vi "removeDuplicates.vi"(8 "error in (no error)":errorcluster, 10 "times":dbl[](array[numeric]) format="%#_18g", 11 "ScriptEventList in":refnum<class "ScriptEventList.lvclass">) -> (0 "error out":errorcluster, 2 "times out":dbl[](array[numeric]) format="%#_8g", 3 "ScriptEventList out":refnum<class "ScriptEventList.lvclass">)   [LabVIEW 2009, in "Tools.lvlib" / "Scripting.lvlib" / "ScriptEventList.lvclass"]
uses:
  ScriptEventList.lvclass
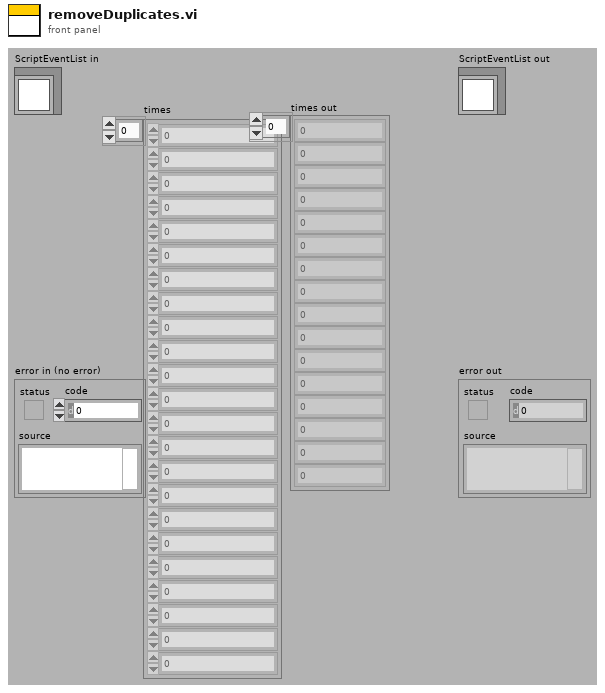
[diagram p1: front panel]
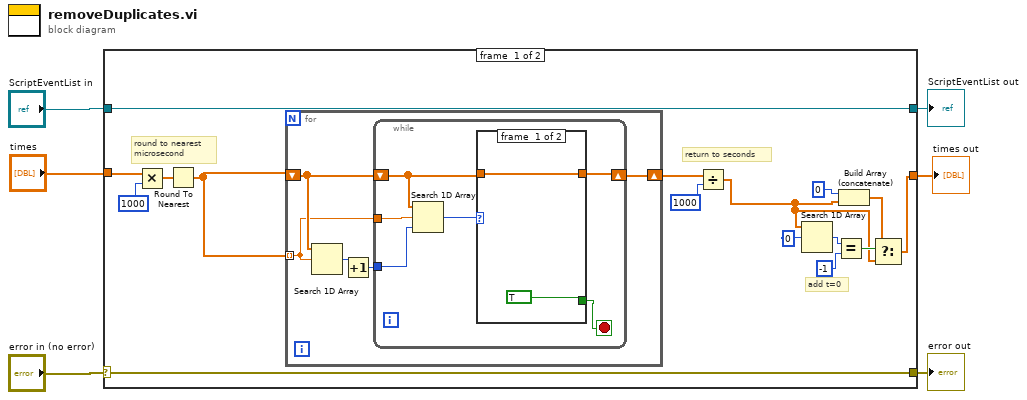
[diagram p0: block diagram]
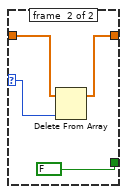
[diagram p2: hidden frame]
diagram:
  n1 = case shown="No Error" "error in (no error)" {
    selector: "error in (no error)" -> [w21 w41]
    tunnel: [w21 w41] -> w5
    tunnel: [w22 w40] -> w3
    tunnel: "ScriptEventList in" -> [w22 w40]
    tunnel: "times" -> [w20 _]
    tunnel: [w7 _] -> w1
    frame #0 {
      # "add t=0"
      # "return to seconds"
      # "round to nearest\nmicrosecond"
      n2 = Multiply(x=w20, y=1000) -> (x*y=w18:dbl[])
      n3 = Round To Nearest(number=w18) -> (nearest integer value=w17:dbl[])
      n4 = for {
        shift-right: [w27] -> w16
        shift-left: w17 -> [w24]
        tunnel: w17 -> [w23] mode=indexing
        n5 = Search 1D Array(1D array=w24, element=w23) -> (index of element=w26:i32)  [unwired: 1 in]
        n6 = Increment(x=w26) -> (x+1=w25:i32)
        n7 = while {
          shift-right: [w31] -> w27
          shift-left: w24 -> [w29]
          tunnel: w25 -> [w30]
          tunnel: w23 -> [w28]
          stop <- w32 stop-if-true
          n8 = Search 1D Array(1D array=w29, element=w28, start index (0)=w30) -> (index of element=w33:i32)
          n9 = case shown="-1" w33 {
            selector: w33 -> [_ w38]
            tunnel: [TRUE FALSE] -> w32
            tunnel: w29 -> [w34 w37]
            tunnel: [w34 w36] -> w31
            frame #0 {
            }
            frame #1 {
              n10 = Delete From Array(array=w37, index=w38) -> (array with subset deleted=w36:dbl[])  [unwired: 1 in, 1 out]
            }
          }
        }
      }
      n11 = Divide(x=w16, y=1000) -> (x/y=w8:dbl[])
      n12 = Search 1D Array(1D array=w8, element=0) -> (index of element=w13:i32)  [unwired: 1 in]
      n13 = Equal?(x=w13, y=-1) -> (x = y?=w11:bool)
      n14 = Build Array (concatenate)(0, w8) -> (w9:dbl[])
      n15 = Select(t=w9, s=w11, f=w8) -> (s? t:f=w7:dbl[])
    }
    frame #1 {
    }
  }
  "error out" <- w5
  "ScriptEventList out" <- w3
  "times out" <- w1
